vi "VelocityProfile.vi"(0 "t":dbl, 1 "a1":dbl=10.0, 3 "a3":dbl=15.0, 5 "s":dbl, 7 "intervalo":dbl=0.016, 9 "v_est":dbl, 11 "v_max":dbl=3.0, 12 "v3":dbl, 13 "s3":dbl) -> (4 "Velocity":dbl, 6 "VelocityProfileState Out":T1, 8 "Velocities":dbl[](array[numeric]), 10 "Time":dbl[](array[numeric]))   [LabVIEW 2017]
uses:
  Controle/VelocityProfileState.ctl
panel:
  in  "Amax":dbl=8.0
  out "NeedMoreAccel":bool
  out "Amin 2":dbl
  out "Amin":dbl
  in  "Reset":bool
  out "Velocity Profile":cluster{dbl[], dbl[]}(graph)
  in  "Tolerancia Vel":dbl=0.01
  in  "Tolerancia Pos":dbl=0.010000000000000004
  out "VelocityProfileState In":T1={"t0"=0.0, "t1"=0.0, "t2"=0.0, "t3"=0.0, "v0"=0.0, "v_max"=3.0, "v3"=0.0, "v2"=0.0, "v1"=0.0, "perfil"=enum."Triangular", "regiao"=0, "s0"=0.0, "s1"=0.0, "s2"=0.0, "v"=0.0, "t"=0.0, "a1"=10.0, "s3"=0.0, "Reset"=FALSE, "s"=0.0, "a3"=15.0, "Ré"=FALSE, "Impossível"=FALSE, "intervalo"=0.0}
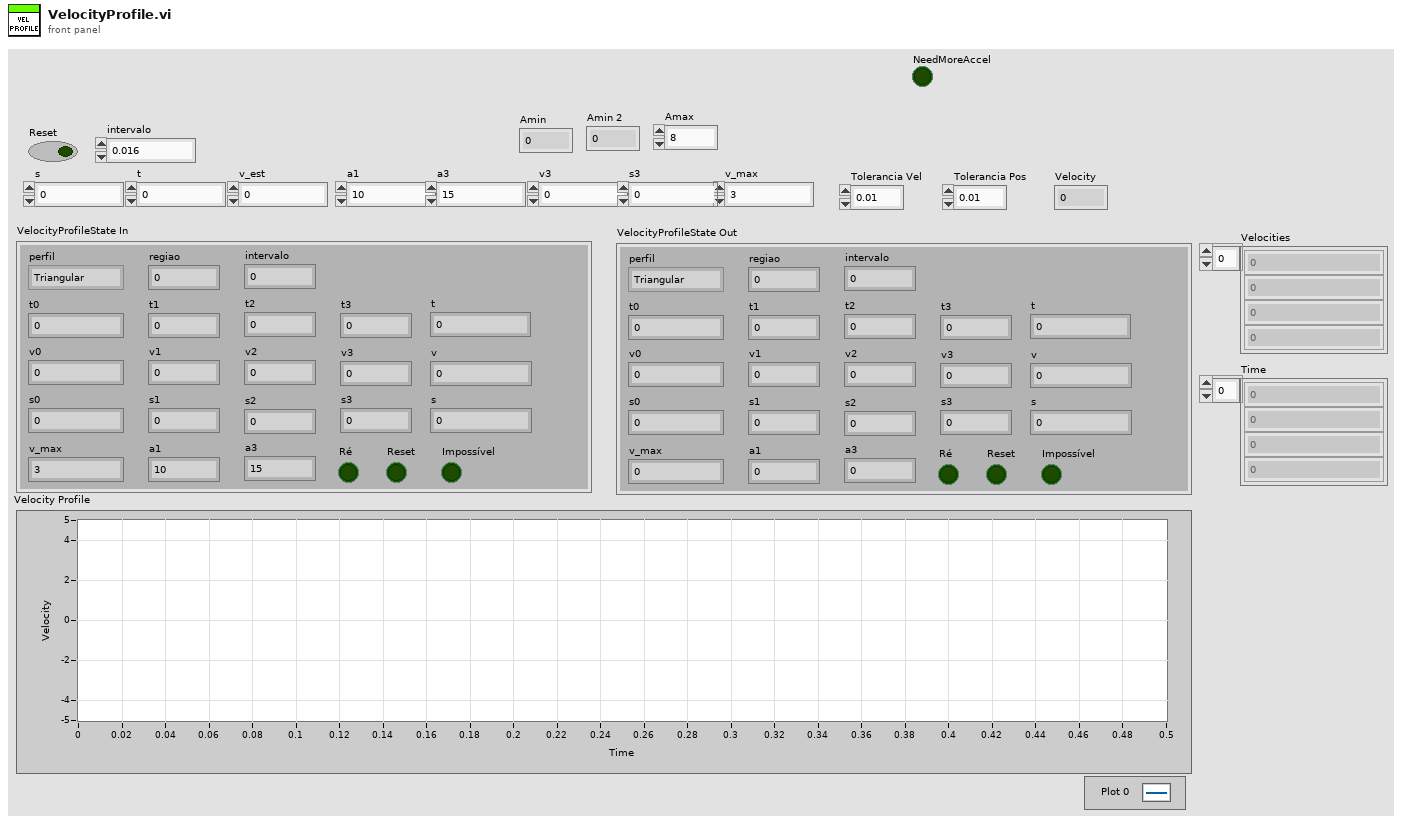
[diagram p1: front panel]
types:
  T1 = typedef "VelocityProfileState.ctl" = cluster{"t0":dbl, "t1":dbl, "t2":dbl, "t3":dbl, "v0":dbl, "v_max":dbl, "v3":dbl, "v2":dbl, "v1":dbl, "perfil":enum16{"Triangular", "Trapezoidal"}, "regiao":i32, "s0":dbl, "s1":dbl, "s2":dbl, "v":dbl, "t":dbl, "a1":dbl, "s3":dbl, "Reset":bool, "s":dbl, "a3":dbl, "Ré":bool, "Impossível":bool, "intervalo":dbl}
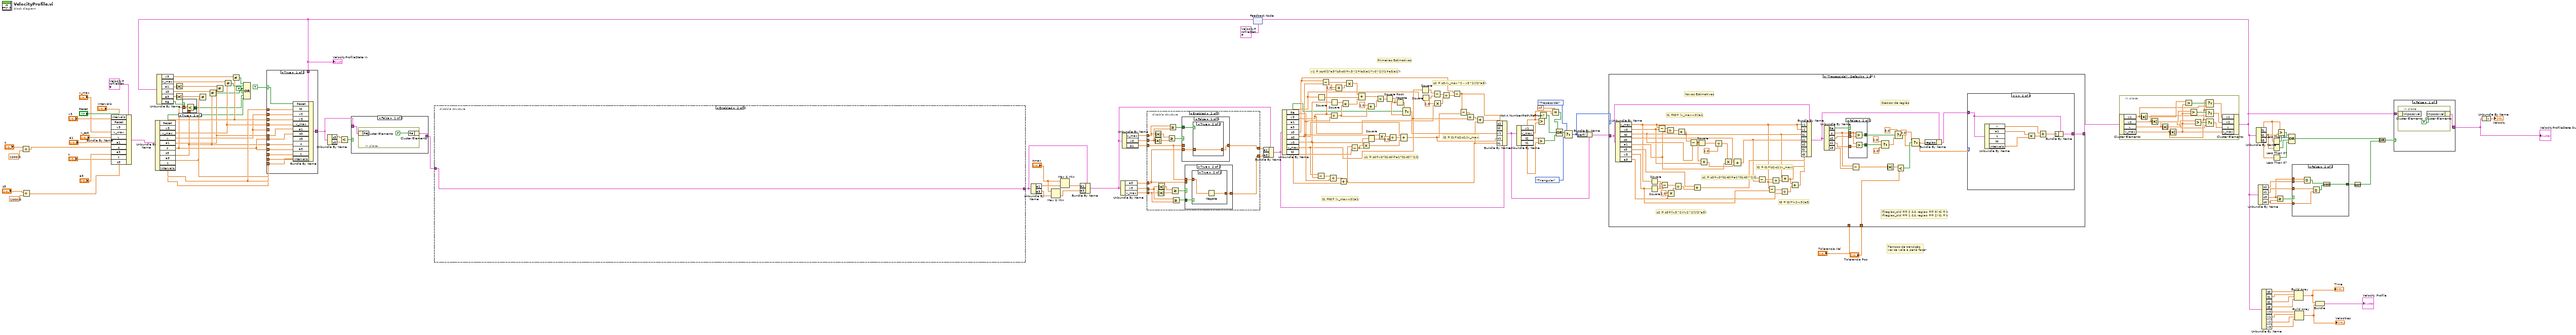
[diagram p0: block diagram]
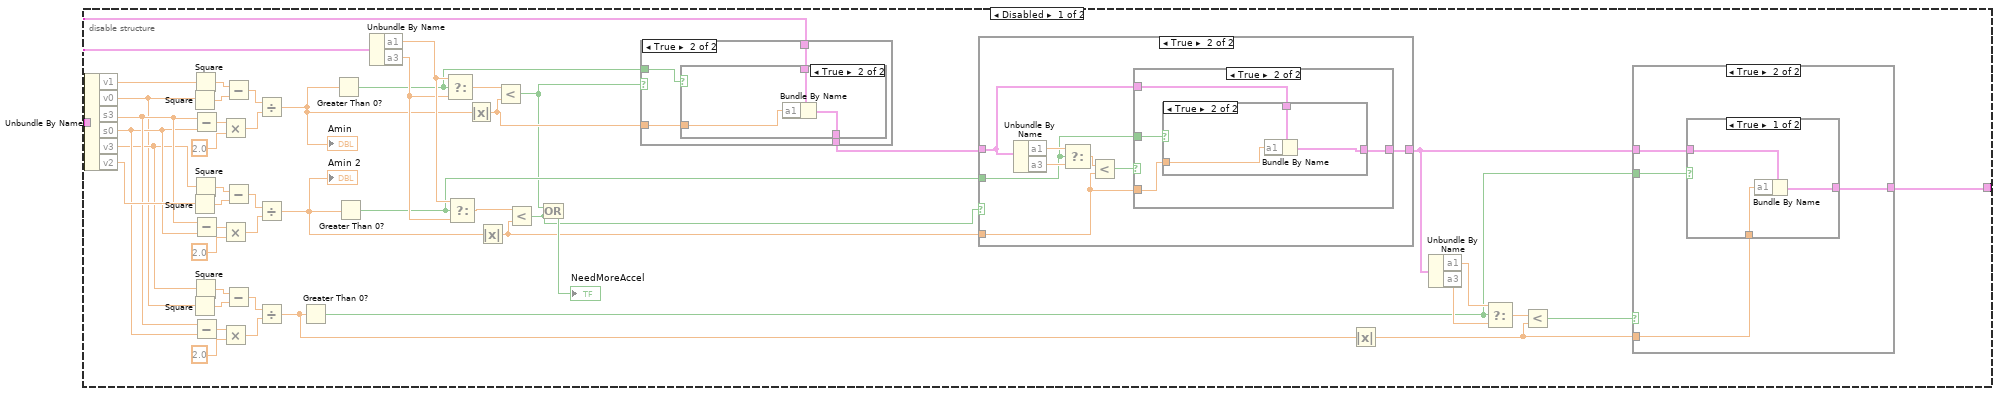
[diagram p2: hidden frame]
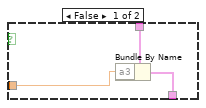
[diagram p4: hidden frame]
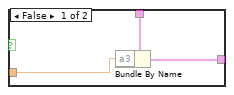
[diagram p7: hidden frame]
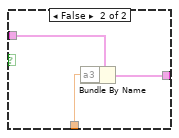
[diagram p9: hidden frame]
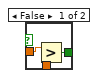
[diagram p10: hidden frame]
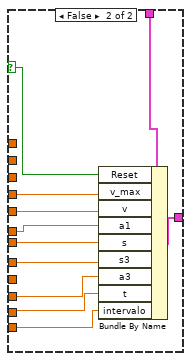
[diagram p11: hidden frame]
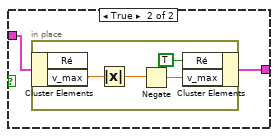
[diagram p12: hidden frame]
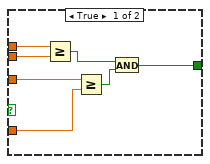
[diagram p13: hidden frame]
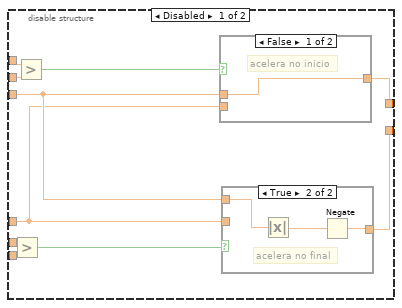
[diagram p14: hidden frame]
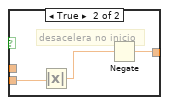
[diagram p16: hidden frame]
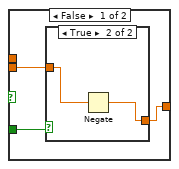
[diagram p17: hidden frame]
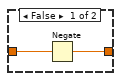
[diagram p20: hidden frame]
diagram:
  w30 = FALSE ("value")
  # "Tempos de transição\nver se vale a pena fazer"
  # "Primeiras Estimativas"
  # "t2 = t1+(s2-s1)/v_max;"
  # "s2 = s3-(v_max^2 - v3^2)/(2*a3);"
  # "s1 = s0+v0*(t1-t0)+a1*(t1-t0)^2/2;"
  # "t1 =t0+ (v_max-v0)/a1;"
  # "v1 = sqrt((2*a3*(s3-s0)+v3^2+(a3/a1)*v0^2)/(1+a3/a1));"
  n1 = Divide(x="s", y=1000.0) -> (x/y=w44:dbl)
  n2 = Divide(x="s3", y=1000.0) -> (x/y=w41:dbl)
  n3 = Bundle By Name(cluster=T1 {"t0"=0.0, "t1"=0.0, "t2"=0.0, "t3"=0.0, "v0"=0.0, "v_max"=0.0, "v3"=0.0, "v2"=0.0, "v1"=0.0, "perfil"=enum."Triangular", "regiao"=0, "s0"=0.0, "s1"=0.0, "s2"=0.0, "v"=0.0, "t"=0.0, "a1"=0.0, "s3"=0.0, "Reset"=FALSE, "s"=0.0, "a3"=0.0, "Ré"=FALSE, "Impossível"=FALSE, "intervalo"=0.0} ("VelocityProfileState In"), "intervalo"="intervalo", "Reset"="Reset", "v3"="v3", "v_max"="v_max", "v"="v_est", "a1"="a1", "s"=w44, "a3"="a3", "t"="t", "s3"=w41) -> (w36:T1)
  n4 = Unbundle By Name(w36) -> ("Reset"=w32:bool, "v3"=w134:dbl, "v_max"=w132:dbl, "v"=w62:dbl, "a1"=w61:dbl, "s"=w34:dbl, "s3"=w33:dbl, "a3"=w66:dbl, "t"=w63:dbl, "intervalo"=w23:dbl)
  n5 = feedback #1(T1 {"t0"=0.0, "t1"=0.0, "t2"=0.0, "t3"=0.0, "v0"=0.0, "v_max"=0.0, "v3"=0.0, "v2"=0.0, "v1"=0.0, "perfil"=enum."Triangular", "regiao"=0, "s0"=0.0, "s1"=0.0, "s2"=0.0, "v"=0.0, "t"=0.0, "a1"=0.0, "s3"=0.0, "Reset"=FALSE, "s"=0.0, "a3"=0.0, "Ré"=FALSE, "Impossível"=FALSE, "intervalo"=0.0} ("VelocityProfileState In")) -> (w11:T1)
  "VelocityProfileState In" <- w11
  n6 = Unbundle By Name(w11) -> ("v3"=w135:dbl, "v_max"=w133:dbl, "a1"=w39:dbl, "s3"=w131:dbl, "a3"=w38:dbl, "Ré"=w35:bool)
  n7 = Absolute Value(x=w39) -> (abs(x)=w40:dbl)
  n8 = Absolute Value(x=w38) -> (abs(x)=w37:dbl)
  n9 = case shown="True" w35 {
    tunnel: w34 -> [w157 w160]
    tunnel: w33 -> [w156 w159]
    tunnel: [w155 w158] -> w31
    frame False {
      n10 = Greater?(x=w157, y=w156) -> (0:w155:bool)
    }
    frame True {
      n11 = Less?(x=w160, y=w159) -> (x < y?=w158:bool)
    }
  }
  n12 = Not Equal?(x=w37, y=w66) -> ()  [unwired: 1 out]
  n13 = Not Equal?(x=w131, y=w33) -> (x != y?=w128:bool)
  n14 = Not Equal?(x=w40, y=w61) -> ()  [unwired: 1 out]
  n15 = Not Equal?(x=w133, y=w132) -> (x != y?=w129:bool)
  n16 = Not Equal?(x=w135, y=w134) -> (x != y?=w130:bool)
  n17 = Compound Arithmetic op=OR(w130, w129, w30, w128, w30, w31, w32) -> ()  [unwired: 1 out]
  n18 = case shown="True" TRUE {
    selector: TRUE -> [w168 w181]
    tunnel: w63 -> [w174 _]
    tunnel: w62 -> [w173 _]
    tunnel: w134 -> [w172 _]
    tunnel: w132 -> [w171 w185]
    tunnel: w62 -> [_ w184]
    tunnel: [w170 w183] -> w152
    tunnel: w11 -> [w169 w182]
    tunnel: w66 -> [w167 w180]
    tunnel: w63 -> [w166 w179]
    tunnel: w34 -> [w165 _]
    tunnel: w61 -> [w161 w178]
    tunnel: w34 -> [w164 w177]
    tunnel: w33 -> [w163 w176]
    tunnel: w23 -> [w162 w175]
    frame True {
      n19 = Bundle By Name(cluster=w169, "Reset"=w168, "t0"=w174, "v0"=w173, "v3"=w172, "v_max"=w171, "a1"=w161, "s0"=w164, "s3"=w163, "s"=w165, "a3"=w167, "t"=w166, "intervalo"=w162) -> (w170:T1)
    }
    frame False {
      n20 = Bundle By Name(cluster=w182, "Reset"=w181, "v_max"=w185, "v"=w184, "a1"=w178, "s"=w177, "s3"=w176, "a3"=w180, "t"=w179, "intervalo"=w175) -> (w183:T1)
    }
  }
  n21 = Unbundle By Name(w152) -> ("s3"=w154:dbl, "s0"=w153:dbl)
  n22 = Less?(x=w154, y=w153) -> (x < y?=w65:bool)
  n23 = case shown="False" w65 {
    tunnel: w152 -> [w187 w190]
    tunnel: [w186 w189] -> w8
    frame False {
      n24 = in-place {
        n25 = in-place-cluster #2(w187) -> ()  [unwired: 1 out]
        n26 = in-place-cluster #2("Ré"=FALSE) -> (w186:T1)
      }
    }
    frame True {
      n27 = in-place {
        n28 = in-place-cluster #3(w190) -> ("v_max"=w194:dbl)  [unwired: 1 out]
        n29 = Absolute Value(x=w194) -> (abs(x)=w193:dbl)
        n30 = Negate(x=w193) -> (-x=w192:dbl)
        n31 = in-place-cluster #3("Ré"=TRUE, "v_max"=w192) -> (w189:T1)
      }
    }
  }
  n32 = disable-structure shown="Enabled" {
    disable-tunnel: w8 -> [w217 w285]
    disable-tunnel: [w198 w285] -> w6
    frame Disabled {
      n33 = Unbundle By Name(w217) -> ("v1"=w230:dbl, "v0"=w207:dbl, "s3"=w210:dbl, "s0"=w209:dbl, "v3"=w208:dbl, "v2"=w229:dbl)
      n34 = Square(x=w207) -> (x^2=w239:dbl)
      n35 = Square(x=w229) -> (x^2=w234:dbl)
      n36 = Square(x=w207) -> (x^2=w213:dbl)
      n37 = Square(x=w230) -> (x^2=w240:dbl)
      n38 = Square(x=w208) -> (x^2=w233:dbl)
      n39 = Square(x=w208) -> (x^2=w214:dbl)
      n40 = Subtract(x=w210, y=w209) -> (x-y=w242:dbl)
      n41 = Subtract(x=w210, y=w209) -> (x-y=w231:dbl)
      n42 = Subtract(x=w210, y=w209) -> (x-y=w216:dbl)
      n43 = Multiply(x=w242, y=2.0) -> (x*y=w237:dbl)
      n44 = Multiply(x=w231, y=2.0) -> (x*y=w236:dbl)
      n45 = Multiply(x=w216, y=2.0) -> (x*y=w211:dbl)
      n46 = Subtract(x=w240, y=w239) -> (x-y=w238:dbl)
      n47 = Subtract(x=w233, y=w234) -> (x-y=w235:dbl)
      n48 = Subtract(x=w214, y=w213) -> (x-y=w212:dbl)
      n49 = Divide(x=w238, y=w237) -> (x/y=w225:dbl)
      "Amin" <- w225
      n50 = Divide(x=w235, y=w236) -> (x/y=w223:dbl)
      "Amin 2" <- w223
      n51 = Divide(x=w212, y=w211) -> (x/y=w203:dbl)
      n52 = Greater Than 0?(x=w203) -> (x > 0?=w201:bool)
      n53 = Greater Than 0?(x=w225) -> (x > 0?=w221:bool)
      n54 = Greater Than 0?(x=w223) -> (x > 0?=w219:bool)
      n55 = Unbundle By Name(w217) -> ("a1"=w228:dbl, "a3"=w227:dbl)
      n56 = Select(t=w228, s=w221, f=w227) -> (s? t:f=w226:dbl)
      n57 = Select(t=w228, s=w219, f=w227) -> (s? t:f=w224:dbl)
      n58 = Absolute Value(x=w225) -> (abs(x)=w220:dbl)
      n59 = Absolute Value(x=w223) -> (abs(x)=w218:dbl)
      n60 = Less?(x=w226, y=w220) -> (x < y?=w196:bool)
      n61 = Less?(x=w224, y=w218) -> (x < y?=w195:bool)
      n62 = Or(x=w196, y=w195) -> (x .or. y?=→"NeedMoreAccel":bool)
      n63 = case shown="True" w196 {
        tunnel: w221 -> [_ w247]
        tunnel: w220 -> [_ w246]
        tunnel: w217 -> [w243 w245]
        tunnel: [w243 w244] -> w197
        frame False {
        }
        frame True {
          n64 = case shown="True" w247 {
            tunnel: w245 -> [w250 w253]
            tunnel: w246 -> [w249 w252]
            tunnel: [w248 w251] -> w244
            frame False {
              n65 = Bundle By Name(cluster=w250, "a3"=w249) -> (w248:T1)
            }
            frame True {
              n66 = Bundle By Name(cluster=w253, "a1"=w252) -> (w251:T1)
            }
          }
        }
      }
      n67 = case shown="True" w195 {
        tunnel: w219 -> [_ w256]
        tunnel: w218 -> [_ w259]
        tunnel: [w254 w258] -> w199
        tunnel: w197 -> [w254 w255]
        frame False {
        }
        frame True {
          n68 = Unbundle By Name(w255) -> ("a1"=w262:dbl, "a3"=w261:dbl)
          n69 = Select(t=w262, s=w256, f=w261) -> (s? t:f=w260:dbl)
          n70 = Less?(x=w260, y=w259) -> (x < y?=w257:bool)
          n71 = case shown="True" w257 {
            tunnel: w259 -> [_ w267]
            tunnel: w255 -> [w263 w266]
            tunnel: [w263 w265] -> w258
            tunnel: w256 -> [_ w264]
            frame False {
            }
            frame True {
              n72 = case shown="True" w264 {
                tunnel: w266 -> [w270 w273]
                tunnel: w267 -> [w269 w272]
                tunnel: [w268 w271] -> w265
                frame False {
                  n73 = Bundle By Name(cluster=w270, "a3"=w269) -> (w268:T1)
                }
                frame True {
                  n74 = Bundle By Name(cluster=w273, "a1"=w272) -> (w271:T1)
                }
              }
            }
          }
        }
      }
      n75 = Absolute Value(x=w203) -> (abs(x)=w200:dbl)
      n76 = Unbundle By Name(w199) -> ("a1"=w206:dbl, "a3"=w205:dbl)
      n77 = Select(t=w206, s=w201, f=w205) -> (s? t:f=w204:dbl)
      n78 = Less?(x=w204, y=w200) -> (x < y?=w202:bool)
      n79 = case shown="True" w202 {
        tunnel: w199 -> [w274 w278]
        tunnel: w201 -> [_ w277]
        tunnel: w200 -> [_ w276]
        tunnel: [w274 w275] -> w198
        frame False {
        }
        frame True {
          n80 = case shown="True" w277 {
            tunnel: w278 -> [w281 w284]
            tunnel: w276 -> [w280 w283]
            tunnel: [w279 w282] -> w275
            frame True {
              n81 = Bundle By Name(cluster=w281, "a1"=w280) -> (w279:T1)
            }
            frame False {
              n82 = Bundle By Name(cluster=w284, "a3"=w283) -> (w282:T1)
            }
          }
        }
      }
    }
    frame Enabled {
    }
  }
  n83 = Unbundle By Name(w6) -> ("a1"=w5:dbl, "a3"=w2:dbl)
  n84 = Max & Min(x="Amax", y=w2) -> (min(x,y)=w1:dbl)  [unwired: 1 out]
  n85 = Max & Min(x="Amax", y=w5) -> (min(x,y)=w4:dbl)  [unwired: 1 out]
  n86 = Bundle By Name(cluster=w6, "a1"=w4, "a3"=w1) -> (w7:T1)
  n87 = Unbundle By Name(w7) -> ("a3"=w67:dbl, "v3"=w112:dbl, "v_max"=w113:dbl)
  n88 = Unbundle By Name(w7) -> ("v_max"=w151:dbl, "v0"=w150:dbl, "a1"=w68:dbl)
  n89 = disable-structure shown="Enabled" {
    disable-tunnel: w151 -> [w295 w315]
    disable-tunnel: w150 -> [w294 w314]
    disable-tunnel: w113 -> [w293 w306]
    disable-tunnel: w112 -> [w292 w307]
    disable-tunnel: [w290 w313] -> w70
    disable-tunnel: [w288 w308] -> w69
    disable-tunnel: w68 -> [w287 w305]
    disable-tunnel: w67 -> [w286 w304]
    frame Disabled {
      n90 = Greater?(x=w292, y=w293) -> (0:w289:bool)
      n91 = Greater?(x=w295, y=w294) -> (0:w291:bool)
      n92 = case shown="False" w291 {
        tunnel: [w300 w302] -> w290
        tunnel: w287 -> [w300 _]
        tunnel: w286 -> [_ w303]
        frame False {
          # "acelera no inicio"
        }
        frame True {
          # "desacelera no inicio"
          n93 = Absolute Value(x=w303) -> (abs(x)=w301:dbl)
          n94 = Negate(x=w301) -> (-x=w302:dbl)
        }
      }
      n95 = case shown="True" w289 {
        tunnel: [w296 w299] -> w288
        tunnel: w287 -> [_ w297]
        tunnel: w286 -> [w296 _]
        frame False {
          # "desacelera no final"
        }
        frame True {
          # "acelera no final"
          n96 = Absolute Value(x=w297) -> (abs(x)=w298:dbl)
          n97 = Negate(x=w298) -> (-x=w299:dbl)
        }
      }
    }
    frame Enabled {
      n98 = Absolute Value(x=w314) -> (abs(x)=w318:dbl)
      n99 = Absolute Value(x=w315) -> (abs(x)=w319:dbl)
      n100 = Absolute Value(x=w306) -> (abs(x)=w310:dbl)
      n101 = Absolute Value(x=w307) -> (abs(x)=w309:dbl)
      n102 = Greater Or Equal?(x=w319, y=w318) -> (x >= y?=w317:bool)
      n103 = Greater Or Equal?(x=w315, y=w314) -> (x >= y?=w316:bool)
      n104 = Greater Or Equal?(x=w309, y=w310) -> (x >= y?=w311:bool)
      n105 = Greater Or Equal?(x=w307, y=w306) -> (x >= y?=w312:bool)
      n106 = case shown="False" w317 {
        tunnel: w305 -> [_ w338]
        tunnel: w316 -> [w334 w340]
        tunnel: [w333 w339] -> w313
        tunnel: w304 -> [w332 _]
        frame False {
          n107 = case shown="True" w334 {
            tunnel: [w335 w337] -> w333
            tunnel: w332 -> [w336 w337]
            frame False {
              n108 = Negate(x=w336) -> (-x=w335:dbl)
            }
            frame True {
            }
          }
        }
        frame True {
          n109 = case shown="True" w340 {
            tunnel: [w341 w343] -> w339
            tunnel: w338 -> [w342 w343]
            frame False {
              n110 = Negate(x=w342) -> (-x=w341:dbl)
            }
            frame True {
            }
          }
        }
      }
      n111 = case shown="True" w311 {
        tunnel: w312 -> [w322 w328]
        tunnel: [w321 w327] -> w308
        tunnel: w305 -> [_ w326]
        tunnel: w304 -> [w320 _]
        frame False {
          n112 = case shown="True" w322 {
            tunnel: [w323 w324] -> w321
            tunnel: w320 -> [w323 w325]
            frame False {
            }
            frame True {
              n113 = Negate(x=w325) -> (-x=w324:dbl)
            }
          }
        }
        frame True {
          n114 = case shown="True" w328 {
            tunnel: [w329 w331] -> w327
            tunnel: w326 -> [w329 w330]
            frame False {
            }
            frame True {
              n115 = Negate(x=w330) -> (-x=w331:dbl)
            }
          }
        }
      }
    }
  }
  n116 = Bundle By Name(cluster=w7, "a1"=w70, "a3"=w69) -> (w71:T1)
  n117 = Unbundle By Name(w71) -> ("Ré"=w64:bool, "v3"=w86:dbl, "a1"=w104:dbl, "a3"=w83:dbl, "s3"=w80:dbl, "s0"=w103:dbl, "v0"=w102:dbl, "v_max"=w78:dbl, "t0"=w111:dbl)
  n118 = Subtract(x=w78, y=w102) -> (x-y=w149:dbl)
  n119 = Square(x=w86) -> (x^2=w99:dbl)
  n120 = Subtract(x=w80, y=w103) -> (x-y=w98:dbl)
  n121 = Divide(x=w149, y=w104) -> (x/y=w148:dbl)
  n122 = Divide(x=w83, y=w104) -> (x/y=w92:dbl)
  n123 = Square(x=w102) -> (x^2=w101:dbl)
  n124 = Multiply(x=2.0, y=w83) -> (x*y=w97:dbl)
  n125 = Add(x=w148, y=w111) -> (x+y=w76:dbl)
  n126 = Multiply(x=w101, y=w92) -> (x*y=w100:dbl)
  n127 = Multiply(x=w98, y=w97) -> (x*y=w95:dbl)
  n128 = Subtract(x=w76, y=w111) -> (x-y=w110:dbl)
  n129 = Compound Arithmetic op=ADD(w95, w99, w100) -> (w94:dbl)
  n130 = Multiply(x=w102, y=w110) -> (x*y=w105:dbl)
  n131 = Add(x=1.0, y=w92) -> (x+y=w93:dbl)
  n132 = Square(x=w110) -> (x^2=w109:dbl)
  n133 = Divide(x=w94, y=w93) -> (x/y=w90:dbl)
  n134 = Multiply(x=w104, y=w109) -> (x*y=w108:dbl)
  n135 = Square Root(x=w90) -> (sqrt(x)=w89:dbl)
  n136 = Divide(x=w108, y=2.0) -> (x/y=w106:dbl)
  n137 = Negate(x=w89) -> (-x=w116:dbl)
  n138 = Compound Arithmetic op=ADD(w103, w106, w105) -> (w72:dbl)
  n139 = Select(t=w116, s=w64, f=w89) -> (s? t:f=w73:dbl)
  n140 = Square(x=w78) -> (x^2=w88:dbl)
  n141 = Square(x=w86) -> (x^2=w87:dbl)
  n142 = Subtract(x=w88, y=w87) -> (x-y=w85:dbl)
  n143 = Multiply(x=2.0, y=w83) -> (x*y=w84:dbl)
  n144 = Divide(x=w85, y=w84) -> (x/y=w81:dbl)
  n145 = Subtract(x=w80, y=w81) -> (x-y=w75:dbl)
  n146 = Subtract(x=w75, y=w72) -> (x-y=w79:dbl)
  n147 = Divide(x=w79, y=w78) -> (x/y=w77:dbl)
  n148 = Add(x=w77, y=w76) -> (x+y=w74:dbl)
  n149 = Bundle By Name(cluster=w71, "s2"=w75, "t2"=w74, "v1"=w73, "s1"=w72, "t1"=w76) -> (w140:T1)
  n150 = Unbundle By Name(w140) -> ("v1"=w27:dbl, "v_max"=w147:dbl, "t2"=w146:dbl, "t1"=w145:dbl)
  n151 = Greater?(x=w146, y=w145) -> (0:w29:bool)
  n152 = Greater?(x=w27, y=w147) -> ()  [unwired: 1 out]
  n153 = Not A Number/Path/Refnum?(number/path/refnum=w27) -> (NaN/Path/Refnum?=w114:bool)
  n154 = Equal?(x=inf, y=w27) -> (x = y?=w28:bool)
  n155 = Compound Arithmetic op=OR(w28, w114, w29) -> (w115:bool)
  n156 = Select(t=enum16{"Triangular", "Trapezoidal"}."Trapezoidal" ("perfil"), s=w115, f=enum16{"Triangular", "Trapezoidal"}."Triangular" ("perfil")) -> (s? t:f=w142:enum16{"Triangular", "Trapezoidal"})
  n157 = Bundle By Name(cluster=w140, "perfil"=w142) -> (w141:T1)
  n158 = case shown="\"Trapezoidal\", Default" w142 {
    tunnel: w141 -> [w396 w456]
    tunnel: [w384 w443] -> w137
    tunnel: "Tolerancia Pos" -> [w367 w441]
    tunnel: "Tolerancia Vel" -> [_ _]
    frame "Trapezoidal", Default {
      # "t3 = t2+(v2-v3)/a3;"
      # "t2 = t1+(s2-s1)/v_max;"
      # "s2 = s3+((v3^2)-(v2^2))/(2*a3);"
      # "s1 = s0+v0*(t1-t0)+a1*(t1-t0)^2/2;"
      # "t1 =t0+ (v_max-v0)/a1;"
      # "if(regiao_old == 2 && regiao == 3) t2 = t;\nif(regiao_old == 1 && regiao == 2) t1 = t;"
      # "Decisor de região"
      # "Novas Estimativas"
      n159 = Unbundle By Name(w396) -> ("v_max"=w349:dbl, "v0"=w361:dbl, "t0"=w371:dbl, "s0"=w360:dbl, "a1"=w370:dbl, "s3"=w351:dbl, "v3"=w347:dbl, "a3"=w354:dbl)
      n160 = Square(x=w349) -> (x^2=w357:dbl)
      n161 = Square(x=w347) -> (x^2=w358:dbl)
      n162 = Subtract(x=w349, y=w361) -> (x-y=w383:dbl)
      n163 = Subtract(x=w358, y=w357) -> (x-y=w356:dbl)
      n164 = Divide(x=w383, y=w370) -> (x/y=w382:dbl)
      n165 = Multiply(x=2.0, y=w354) -> (x*y=w355:dbl)
      n166 = Divide(x=w356, y=w355) -> (x/y=w352:dbl)
      n167 = Add(x=w382, y=w371) -> (x+y=w374:dbl)
      n168 = Subtract(x=w374, y=w371) -> (x-y=w362:dbl)
      n169 = Add(x=w351, y=w352) -> (x+y=w377:dbl)
      n170 = Square(x=w362) -> (x^2=w381:dbl)
      n171 = Multiply(x=w362, y=w361) -> (x*y=w359:dbl)
      n172 = Divide(x=w381, y=2.0) -> (x/y=w379:dbl)
      n173 = Multiply(x=w379, y=w370) -> (x*y=w378:dbl)
      n174 = Compound Arithmetic op=ADD(w360, w378, w359) -> (w376:dbl)
      n175 = Subtract(x=w377, y=w376) -> (x-y=w350:dbl)
      n176 = Subtract(x=w349, y=w347) -> (x-y=w348:dbl)
      n177 = Divide(x=w350, y=w349) -> (x/y=w375:dbl)
      n178 = Divide(x=w348, y=w354) -> (x/y=w372:dbl)
      n179 = Add(x=w374, y=w375) -> (x+y=w373:dbl)
      n180 = Add(x=w373, y=w372) -> (x+y=w369:dbl)
      n181 = Bundle By Name(cluster=w396, "v1"=w349, "v2"=w349, "t1"=w374, "s1"=w376, "s2"=w377, "t2"=w373, "t3"=w369) -> (w387:T1)
      n182 = Unbundle By Name(w387) -> ("Ré"=w346:bool, "s"=w392:dbl, "s2"=w395:dbl, "s1"=w345:dbl, "s3"=w366:dbl)
      n183 = case shown="False" w346 {
        tunnel: w395 -> [w401 w406]
        tunnel: [w400 w405] -> w394
        tunnel: w392 -> [w399 w404]
        tunnel: w345 -> [w398 w403]
        tunnel: [w397 w402] -> w344
        frame True {
          n184 = Less?(x=w399, y=w401) -> (x < y?=w400:bool)
          n185 = Less?(x=w399, y=w398) -> (x < y?=w397:bool)
        }
        frame False {
          n186 = Greater?(x=w404, y=w406) -> (0:w405:bool)
          n187 = Greater?(x=w404, y=w403) -> (0:w402:bool)
        }
      }
      n188 = Subtract(x=w392, y=w366) -> (x-y=w391:dbl)
      n189 = Select(t=2.0, s=w344, f=1.0) -> (s? t:f=w363:dbl)
      n190 = Absolute Value(x=w391) -> (abs(x)=w390:dbl)
      n191 = Select(t=3.0, s=w394, f=w363) -> (s? t:f=w368:dbl)
      n192 = Less?(x=w390, y=w367) -> (x < y?=w389:bool)
      n193 = Select(t=0.0, s=w389, f=w368) -> (s? t:f=w386:dbl)
      n194 = Bundle By Name(cluster=w387, "regiao"=w386) -> (w385:T1)
      n195 = case shown="1" w386 {
        tunnel: w385 -> [w409 w416 w418 w426]
        tunnel: [w407 w415 w419 w425] -> w384
        frame 0, Default {
          n196 = Bundle By Name(cluster=w409, "v"=0.0) -> (w407:T1)
        }
        frame 1 {
          n197 = Unbundle By Name(w416) -> ("v"=w412:dbl, "a1"=w414:dbl, "intervalo"=w410:dbl)  [unwired: 2 out]
          n198 = Multiply(x=w414, y=w410) -> (x*y=w413:dbl)
          n199 = Add(x=w412, y=w413) -> (x+y=w411:dbl)
          n200 = Bundle By Name(cluster=w416, "v"=w411) -> (w415:T1)
        }
        frame 2 {
          n201 = Unbundle By Name(w418) -> ("v_max"=w417:dbl)
          n202 = Bundle By Name(cluster=w418, "v"=w417) -> (w419:T1)
        }
        frame 3 {
          n203 = Unbundle By Name(w426) -> ("v"=w422:dbl, "a3"=w424:dbl, "intervalo"=w420:dbl)  [unwired: 2 out]
          n204 = Multiply(x=w424, y=w420) -> (x*y=w423:dbl)
          n205 = Subtract(x=w422, y=w423) -> (x-y=w421:dbl)
          n206 = Bundle By Name(cluster=w426, "v"=w421) -> (w425:T1)
        }
      }
    }
    frame "Triangular" {
      # "if(regiao_old == 1 && regiao == 3) t1 = t;"
      # "Decisor de região"
      # "Novas Estimativas"
      # "t3 = t1+(v1-v3)/a3;"
      # "s1 = s0+v0*(t1-t0)+a1*(t1-t0)^2/2;"
      # "t1 = t0+(v1-v0)/a1;"
      n207 = Unbundle By Name(w456) -> ("v0"=w429:dbl, "t0"=w462:dbl, "v1"=w433:dbl, "s0"=w459:dbl, "a1"=w436:dbl, "a3"=w435:dbl, "v3"=w432:dbl)
      n208 = Subtract(x=w433, y=w429) -> (x-y=w464:dbl)
      n209 = Subtract(x=w433, y=w432) -> (x-y=w434:dbl)
      n210 = Divide(x=w464, y=w436) -> (x/y=w463:dbl)
      n211 = Add(x=w463, y=w462) -> (x+y=w457:dbl)
      n212 = Divide(x=w434, y=w435) -> (x/y=w458:dbl)
      n213 = Add(x=w457, y=w458) -> (x+y=w431:dbl)
      n214 = Subtract(x=w457, y=w462) -> (x-y=w430:dbl)
      n215 = Multiply(x=w430, y=w429) -> (x*y=w428:dbl)
      n216 = Square(x=w430) -> (x^2=w461:dbl)
      n217 = Divide(x=w461, y=2.0) -> (x/y=w438:dbl)
      n218 = Multiply(x=w438, y=w436) -> (x*y=w437:dbl)
      n219 = Compound Arithmetic op=ADD(w459, w437, w428) -> (w442:dbl)
      n220 = Bundle By Name(cluster=w456, "t1"=w457, "s1"=w442, "v2"=w433, "t2"=w457, "t3"=w431, "s2"=w442) -> (w446:T1)
      n221 = Unbundle By Name(w446) -> ("Ré"=w427:bool, "s"=w452:dbl, "s1"=w455:dbl, "s3"=w451:dbl)
      n222 = case shown="True" w427 {
        tunnel: w455 -> [w467 w468]
        tunnel: [w466 w470] -> w454
        tunnel: w452 -> [w465 w469]
        frame False {
          n223 = Greater?(x=w465, y=w467) -> (0:w466:bool)
        }
        frame True {
          n224 = Less?(x=w469, y=w468) -> (x < y?=w470:bool)
        }
      }
      n225 = Subtract(x=w452, y=w451) -> (x-y=w450:dbl)
      n226 = Select(t=3.0, s=w454, f=1.0) -> (s? t:f=w448:dbl)
      n227 = Absolute Value(x=w450) -> (abs(x)=w449:dbl)
      n228 = Less?(x=w449, y=w441) -> (x < y?=w447:bool)
      n229 = Select(t=0.0, s=w447, f=w448) -> (s? t:f=w445:dbl)
      n230 = Bundle By Name(cluster=w446, "regiao"=w445) -> (w444:T1)
      n231 = case shown="0, Default" w445 {
        tunnel: w444 -> [w473 w480 w487]
        tunnel: [w471 w479 w486] -> w443
        frame 0, Default {
          n232 = Bundle By Name(cluster=w473, "v"=0.0) -> (w471:T1)
        }
        frame 1 {
          n233 = Unbundle By Name(w480) -> ("v"=w476:dbl, "a1"=w478:dbl, "intervalo"=w474:dbl)  [unwired: 2 out]
          n234 = Multiply(x=w478, y=w474) -> (x*y=w477:dbl)
          n235 = Add(x=w476, y=w477) -> (x+y=w475:dbl)
          n236 = Bundle By Name(cluster=w480, "v"=w475) -> (w479:T1)
        }
        frame 3 {
          n237 = Unbundle By Name(w487) -> ("v"=w483:dbl, "a3"=w485:dbl, "intervalo"=w481:dbl)  [unwired: 2 out]
          n238 = Multiply(x=w485, y=w481) -> (x*y=w484:dbl)
          n239 = Subtract(x=w483, y=w484) -> (x-y=w482:dbl)
          n240 = Bundle By Name(cluster=w487, "v"=w482) -> (w486:T1)
        }
      }
    }
  }
  n241 = in-place {
    n242 = in-place-cluster #4(w137) -> ("v1"=w490:dbl, "v2"=w489:dbl, "v"=w488:dbl, "v_max"=w491:dbl)
    n243 = Absolute Value(x=w490) -> (abs(x)=w496:dbl)
    n244 = Absolute Value(x=w489) -> (abs(x)=w495:dbl)
    n245 = Absolute Value(x=w488) -> (abs(x)=w494:dbl)
    n246 = Absolute Value(x=w491) -> (abs(x)=w493:dbl)
    n247 = Greater?(x=w496, y=w493) -> (0:w501:bool)
    n248 = Greater?(x=w495, y=w493) -> (0:w500:bool)
    n249 = Greater?(x=w494, y=w493) -> (0:w492:bool)
    n250 = Select(t=w491, s=w501, f=w490) -> (s? t:f=w499:dbl)
    n251 = Select(t=w491, s=w500, f=w489) -> (s? t:f=w498:dbl)
    n252 = Select(t=w491, s=w492, f=w488) -> (s? t:f=w497:dbl)
    n253 = in-place-cluster #4("v1"=w499, "v2"=w498, "v"=w497, "v_max"=w493) -> (w22:T1)
  }
  n254 = feedback-in #1(w22) -> ()
  n255 = Unbundle By Name(w22) -> ("t1"=w53:dbl, "t2"=w10:dbl, "t3"=w50:dbl)
  n256 = Unbundle By Name(w22) -> ("s2"=w18:dbl, "s1"=w20:dbl, "s3"=w17:dbl, "s0"=w19:dbl)
  n257 = Unbundle By Name(w22) -> ("t0"=w126:dbl, "t1"=w125:dbl, "t2"=w124:dbl, "t3"=w123:dbl, "v0"=w122:dbl, "v1"=w121:dbl, "v2"=w120:dbl, "v3"=w119:dbl)
  n258 = Less Than 0?(x=w53) -> (x < 0?=w52:bool)
  n259 = Less Than 0?(x=w10) -> (x < 0?=w51:bool)
  n260 = Less Than 0?(x=w50) -> (x < 0?=w49:bool)
  n261 = Greater Or Equal?(x=w17, y=w19) -> (x >= y?=w21:bool)
  n262 = Greater?(x=w53, y=w10) -> (0:w9:bool)
  n263 = Compound Arithmetic op=OR(w9, w52, w51, w49) -> (w15:bool)
  n264 = case shown="False" w21 {
    tunnel: w20 -> [w507 w514]
    tunnel: w19 -> [w508 w515]
    tunnel: w18 -> [w506 w513]
    tunnel: w17 -> [w505 w512]
    tunnel: [w502 w509] -> w14
    frame True {
      n265 = Greater Or Equal?(x=w505, y=w506) -> (x >= y?=w503:bool)
      n266 = Greater Or Equal?(x=w507, y=w508) -> (x >= y?=w504:bool)
      n267 = And(x=w503, y=w504) -> (x .and. y?=w502:bool)
    }
    frame False {
      n268 = Less Or Equal?(x=w512, y=w513) -> (x <= y?=w510:bool)
      n269 = Less Or Equal?(x=w514, y=w515) -> (x <= y?=w511:bool)
      n270 = And(x=w510, y=w511) -> (x .and. y?=w509:bool)
    }
  }
  n271 = Build Array(w126, w125, w124, w123) -> (w118:dbl[])
  "Time" <- w118
  n272 = Build Array(w122, w121, w120, w119) -> (w117:dbl[])
  "Velocities" <- w117
  n273 = Bundle(w118, w117) -> (→"Velocity Profile":cluster{dbl[], dbl[]})  [unwired: 1 in]
  n274 = Not(x=w14) -> (.not. x?=w13:bool)
  n275 = Or(x=w15, y=w13) -> (x .or. y?=w16:bool)
  n276 = case shown="False" w16 {
    tunnel: w22 -> [w517 w520]
    tunnel: [w516 w519] -> w48
    frame False {
      n277 = in-place {
        n278 = in-place-cluster #5(w517) -> ()  [unwired: 1 out]
        n279 = in-place-cluster #5("Impossível"=FALSE) -> (w516:T1)
      }
    }
    frame True {
      n280 = in-place {
        n281 = in-place-cluster #6(w520) -> ()  [unwired: 1 out]
        n282 = in-place-cluster #6("Impossível"=TRUE) -> (w519:T1)
      }
    }
  }
  "VelocityProfileState Out" <- w48
  n283 = Unbundle By Name(w48) -> ("v"=→"Velocity":dbl)
